vi "Matrix_LltDecompose.vi"(10 "LowerTriangle":bool, 11 "input matrix":T1) -> (0 "Error":bool, 3 "output Cholesky Decomp":T1)   [LabVIEW 2019, in "Trajectory_Library.lvlib"]
doc: "Creates a new LINEAR SYSTEM data cluster with the specified values. \n\n\nInputs: \n - XXX -- XXX.\n\nOutputs:\n - XXX -- XXX."
uses:
  <vilib>/Analysis/Matrix/Datatypes/RealMatrix.ctl
  Trajectory_Library.lvlib
  <vilib>/Analysis/NI_AALPro.lvlib
  <vilib>/Analysis/7linalg.llb/Real Cholesky Factorization.vi
  <vilib>/Analysis/Matrix/NI_Matrix.lvlib
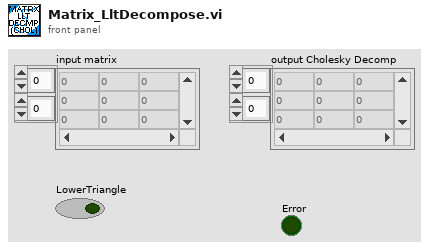
[diagram p1: front panel]
types:
  T1 = typedef "NI_Matrix.lvlib/RealMatrix.ctl" = dbl[][]
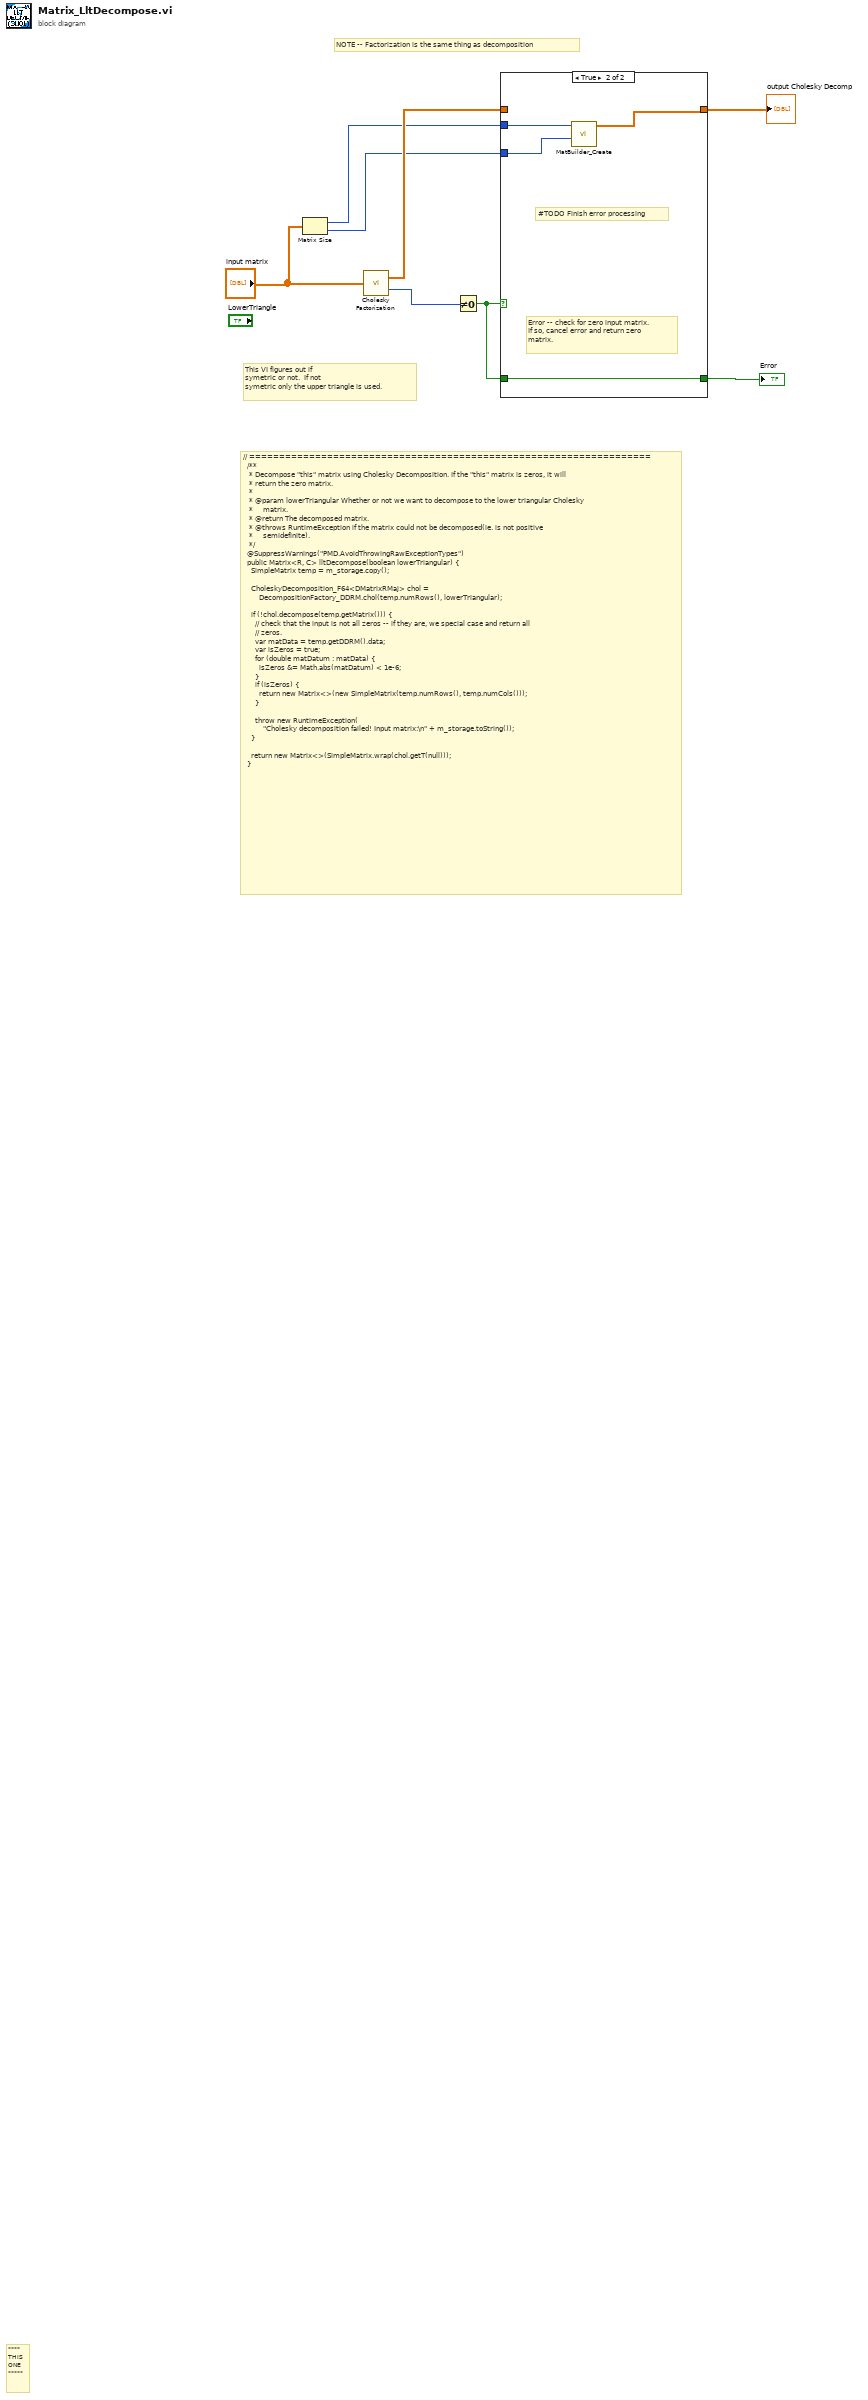
[diagram p0: block diagram]
diagram:
  # "This VI figures out if\nsymetric or not.  If not \nsymetric only the upper triangle is used."
  # "NOTE -- Factorization is the same thing as decomposition"
  # "// ===================================================================\n  /**\n   * Decompose \"this\" matrix using Cholesky Decomposition. If the \"this\" matrix is zeros, it will\n   * return the zero matrix.\n   *\n   * @param lowerTriangular Whether or not we want to decompose to the lower triangular Cholesky\n   *     matrix.\n   * @return The decomposed matrix.\n   * @throws RuntimeException if the matrix could not be decomposed(ie. is not positive\n   *     semidefinite).\n   */\n  @SuppressWarnings(\"PMD.AvoidThrowingRawExceptionTypes\")\n  public Matrix<R, C> lltDecompose(boolean lowerTriangular) {\n    SimpleMatrix temp = m_storage.copy();\n\n    CholeskyDecomposition_F64<DMatrixRMaj> chol =\n        DecompositionFactory_DDRM.chol(temp.numRows(), lowerTriangular);\n\n    if (!chol.decompose(temp.getMatrix())) {\n      // check that the input is not all zeros -- if they are, we special case and return all\n      // zeros.\n      var matData = temp.getDDRM().data;\n      var isZeros = true;\n      for (double matDatum : matData) {\n        isZeros &= Math.abs(matDatum) < 1e-6;\n      }\n      if (isZeros) {\n        return new Matrix<>(new SimpleMatrix(temp.numRows(), temp.numCols()));\n      }\n\n      throw new RuntimeException(\n          \"Cholesky decomposition failed! Input matrix:\\n\" + m_storage.toString());\n    }\n\n    return new Matrix<>(SimpleMatrix.wrap(chol.getT(null)));\n  }"
  # "****\nTHIS\nONE\n*****"
  n1 = Matrix Size(0:"input matrix") -> (1:w2:i32, 2:w1:i32)
  n2 = call-poly <vilib>:"Cholesky Factorization.vi"("A"="input matrix") -> ("Cholesky"=w6:T1, "error"=w7:i32)
  n3 = Not Equal To 0?(x=w7) -> (x != 0?=w4:bool)
  n4 = case shown="True" w4 {
    tunnel: [w10 w12] -> w5
    tunnel: w6 -> [w10 _]
    tunnel: w4 -> [w9 w11]
    tunnel: [w9 w11] -> w3
    tunnel: w2 -> [_ w14]
    tunnel: w1 -> [_ w13]
    frame False {
    }
    frame True {
      # "#TODO Finish error processing"
      # "Error -- check for zero input matrix.\nIf so, cancel error and return zero \nmatrix."
      n5 = call "MatBuilder_Create.vi"("Columns"=w13, "Rows"=w14) -> ("output matrix"=w12:T1)  [unwired: 9 in]
    }
  }
  "output Cholesky Decomp" <- w5
  "Error" <- w3
